vi "createEvents.vi"(8 "error in (no error)":errorcluster, 11 "TCPComEvents in":refnum<class "TCPComEvents.lvclass">) -> (0 "error out":errorcluster, 3 "TCPComEvents out":refnum<class "TCPComEvents.lvclass">)   [LabVIEW 2016, in "TCPComEvents.lvclass"]
uses:
  TCPComEvents.lvclass
  TCPComEvents.lvclass/TCPComEvents.ctl
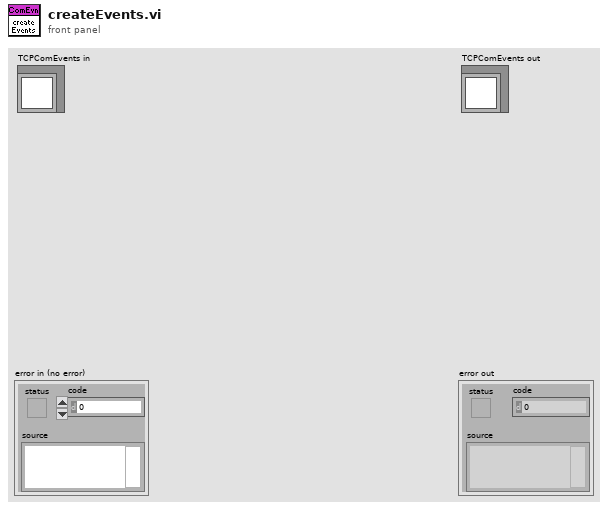
[diagram p1: front panel]
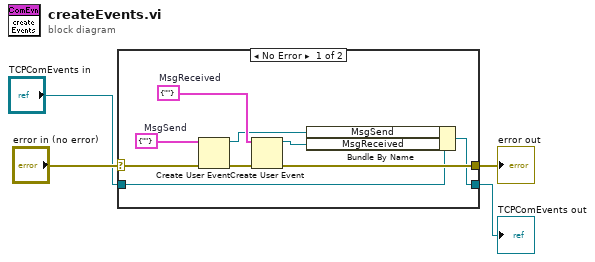
[diagram p0: block diagram]
diagram:
  n1 = case shown="No Error" "error in (no error)" {
    selector: "error in (no error)" -> [w5 w15]
    tunnel: [w13 w15] -> w3
    tunnel: [w8 w14] -> w1
    tunnel: "TCPComEvents in" -> [w9 w14]
    frame No Error {
      w10 = cluster{"message":string} {"message"=""}  # MsgReceived
      w11 = cluster{"message":string} {"message"=""}  # MsgSend
      n2 = Create User Event(user event datatype=w11, error in=w5) -> (user event=w7:refnum<user-event>, error out=w12:errorcluster)
      n3 = Create User Event(user event datatype=w10, error in=w12) -> (user event=w6:refnum<user-event>, error out=w13:errorcluster)
      n4 = Bundle By Name(cluster=w9, "MsgSend"=w7, "MsgReceived"=w6) -> (w8:refnum<class "TCPComEvents.lvclass">)
    }
    frame Error {
    }
  }
  "error out" <- w3
  "TCPComEvents out" <- w1
